vi "CameraReset.vi"(8 "error constant":errorcluster, 10 "Camera Settings":T1={"EM Gain :"=100.0, "Pre Amp Gain :"=1.0, "VS Speed [Index] :"=1.0, "Conv HS Speed :"=1.0, "Exposure Time [s] :"=1.0, "Temperature :"=0.2, "EM HS Speex [s]"=0.0, "Gain > 300 :"=FALSE}) -> (0 "error constant 2":errorcluster)   [LabVIEW 2017]
uses:
  CameraSettings.ctl
  <userlib>/atmcd32d.llb/AcquisitionMode_mode typedef.ctl
  <userlib>/atmcd32d.llb/TriggerMode_mode typedef.ctl
panel:
  out "DLL error code":u32
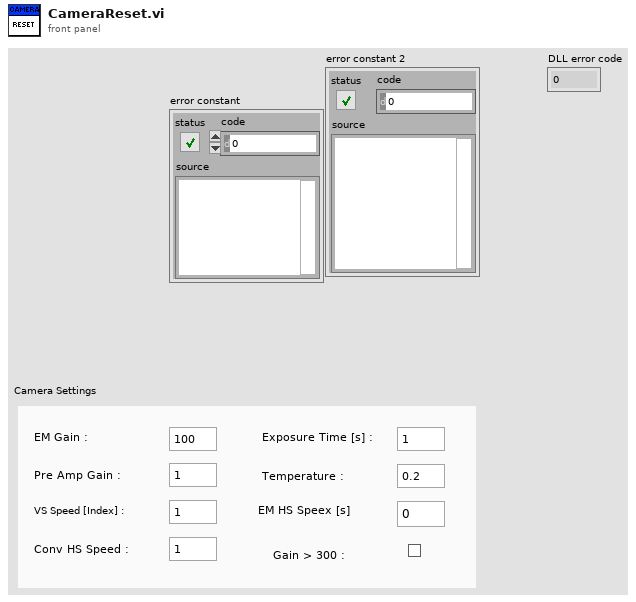
[diagram p1: front panel]
types:
  T1 = typedef "CameraSettings.ctl" = cluster{"EM Gain :":dbl, "Pre Amp Gain :":dbl, "VS Speed [Index] :":dbl, "Conv HS Speed :":dbl, "Exposure Time [s] :":dbl, "Temperature :":dbl, "EM HS Speex [s]":dbl, "Gain > 300 :":bool}
  T2 = typedef "TriggerMode_mode typedef.ctl" = enum16{"Internal", "External", "N/A (2)", "N/A (3)", "N/A (4)", "N/A (5)", "External Start", "External Exposure (Bulb)", "N/A (8)", "External FVB EM", "Software", "N/A (11)", "External Charge Shifting"}
  T3 = typedef "AcquisitionMode_mode typedef.ctl" = enum16{"Reserved (0)", "Single Scan", "Accumulate", "Kinetics", "Fast Kinetics", "Run Till Abort", "Reserved (6)", "Reserved (7)", "Reserved (8)", "Time Delayed Integration"}
  T4 = cluster{"EM gain?":bool, "EM gain":u16, "preamp gain":enum16{"0", "1", "2", "3"}, "VS speed":enum16{"0", "1", "2", "3"}, "conv HS speed":enum16{"0", "1"}, "EM HS speed":enum16{"0", "1", "2", "3"}}
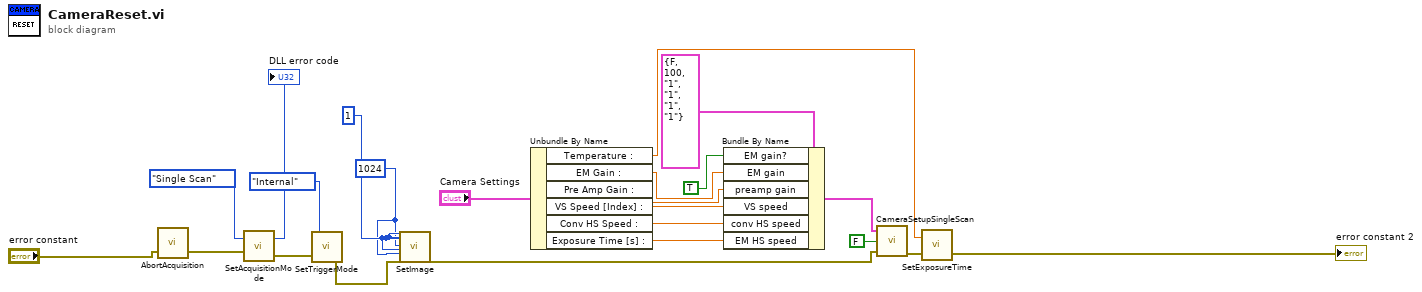
[diagram p0: block diagram]
diagram:
  w5 = 1024 ("hstart")
  w6 = 1 ("vbin")
  n1 = call <userlib>:"AbortAcquisition.vi"("error in (no error)"="error constant") -> ("error out"=w2:errorcluster)  [unwired: 1 in, 1 out]
  n2 = call <userlib>:"SetAcquisitionMode.vi"("error in (no error)"=w2, "mode"=AcquisitionMode_mode_typedef."Single Scan") -> ("error out"=w9:errorcluster, "DLL error code"=→"DLL error code":u32)
  n3 = call <userlib>:"SetTriggerMode.vi"("error in (no error)"=w9, "mode"=TriggerMode_mode_typedef."Internal") -> ("error out"=w7:errorcluster)  [unwired: 1 out]
  n4 = call <userlib>:"SetImage.vi"("hbin"=w6, "vbin"=w6, "hstart"=w6, "hend"=w5, "vstart"=w6, "vend"=w5, "error in (no error)"=w7) -> ("error out"=w4:errorcluster)  [unwired: 19 in, 1 out]
  n5 = Unbundle By Name("Camera Settings") -> ("Temperature :"=w12:dbl, "EM Gain :"=w19:dbl, "Pre Amp Gain :"=w18:dbl, "VS Speed [Index] :"=w17:dbl, "Conv HS Speed :"=w16:dbl, "Exposure Time [s] :"=w15:dbl)
  n6 = Bundle By Name(cluster=T4 {"EM gain?"=FALSE, "EM gain"=100, "preamp gain"=enum."1", "VS speed"=enum."1", "conv HS speed"=enum."1", "EM HS speed"=enum."1"} ("Camera settings"), "EM gain?"=TRUE, "EM gain"=w19, "preamp gain"=w18, "VS speed"=w17, "conv HS speed"=w16, "EM HS speed"=w15) -> (w22:T4)
  n7 = call "CameraSetupSingleScan.vi"("error in (no error)"=w4, "EM adv"=FALSE, "Camera settings"=w22) -> ("error out"=w13:errorcluster)  [unwired: 3 out]
  n8 = call <userlib>:"SetExposureTime.vi"("error in (no error)"=w13, "time"=w12) -> ("error out"=→"error constant 2":errorcluster)  [unwired: 1 out]
